vi "MCA_Confirming Interested area Dialog.vi"(2 "终点道址：":u32=3600, 3 "起点道址：":u32=3600) -> (0 "终点道址： 2":u32=3600, 1 "起点道址： 2":u32=3600)   [LabVIEW 2014]
panel:
  in  "按钮_确定":bool
  # "请确认寻峰所用感兴区边界："
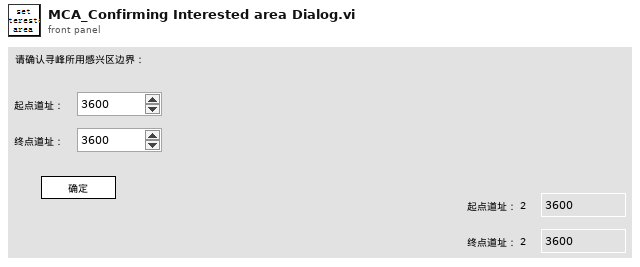
[diagram p1: front panel]
types:
  T1 = typedef "枚举常量_状态机.ctl" = enum16{"初始化", "等待", "完成"}
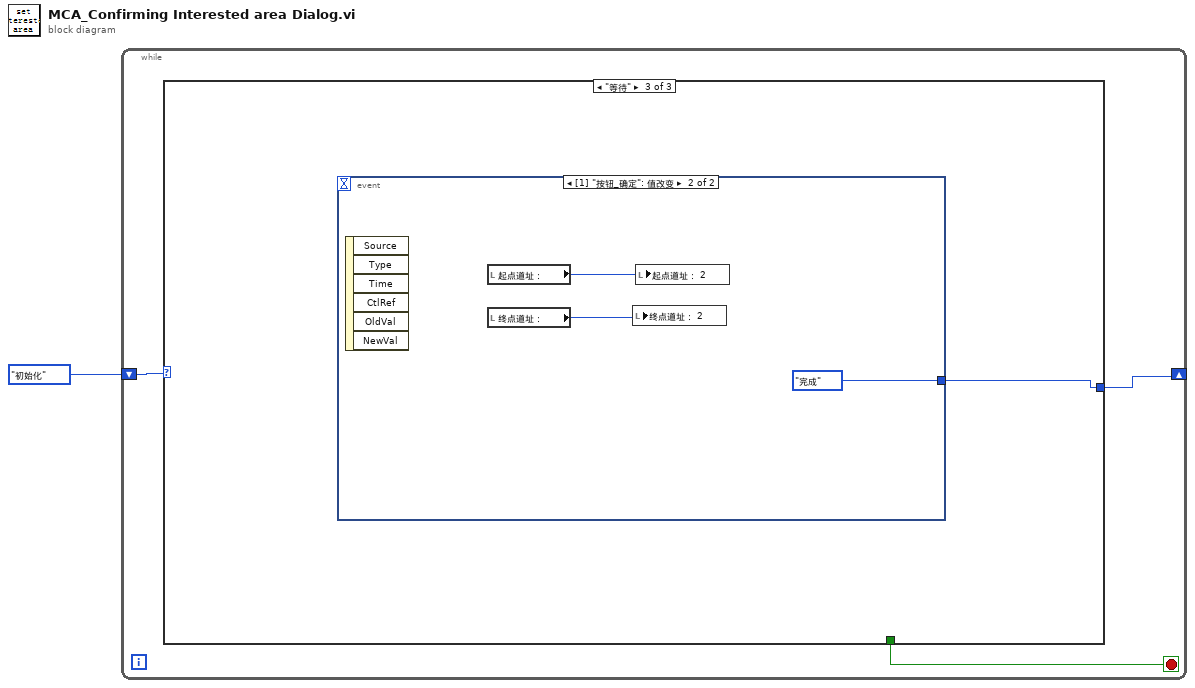
[diagram p0: block diagram]
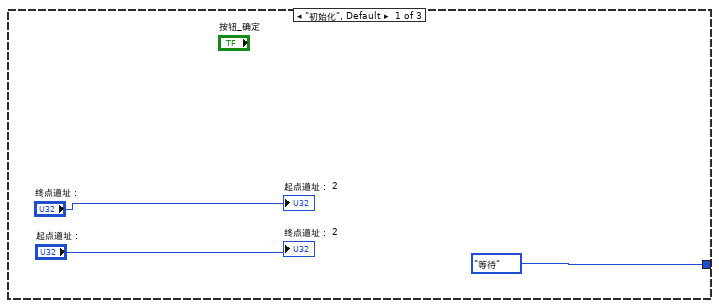
[diagram p2: hidden frame]
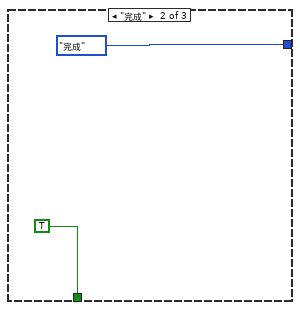
[diagram p3: hidden frame]
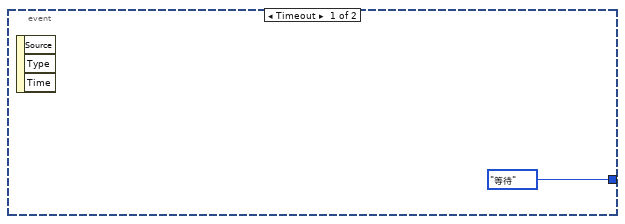
[diagram p4: hidden frame]
diagram:
  n1 = while {
    shift-right: [w3] -> _
    shift-left: 枚举常量_状态机."初始化" ("枚举") -> [w4]
    stop <- w2 stop-if-true
    n2 = case shown="\"等待\"" w4 {
      tunnel: [枚举常量_状态机."等待" ("枚举") 枚举常量_状态机."完成" ("枚举") w10] -> w3
      tunnel: [_ TRUE _] -> w2
      frame "初始化", Default {
        "起点道址： 2" <- "终点道址："
        "终点道址： 2" <- "起点道址："
      }
      frame "完成" {
      }
      frame "等待" {
        n3 = event shown="[1] \"按钮_确定\": 值改变" {
          selector: _ -> [_ _]
          dyn-events: _ -> [_ _]
          timeout: _ -> [_ _]
          tunnel: [枚举常量_状态机."等待" ("枚举") 枚举常量_状态机."完成" ("枚举")] -> w10
          event Timeout {
            n4 = event-data() -> ()  [unwired: 1 in, 3 out]
          }
          event "按钮_确定": Value Change {
            n5 = event-data() -> ()  [unwired: 1 in, 6 out]
            n6 = local read "起点道址："() -> (w13:u32)
            n7 = local read "终点道址："() -> (w12:u32)
            n8 = local write "终点道址： 2"(w12) -> ()
            n9 = local write "起点道址： 2"(w13) -> ()
          }
        }
      }
    }
  }
